vi "Cmd.Echo.vi"(6 "Timeout [ms] (1000)":i32=1000, 8 "error in":errorcluster, 10 "String":string="echoo", 11 "cID in":refnum<k5>) -> (0 "error out":errorcluster, 3 "cID out":refnum<k5>)   [LabVIEW 2016]
panel:
  out "debug":string
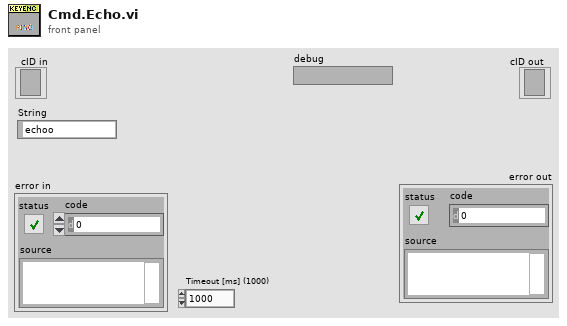
[diagram p1: front panel]
types:
  T1 = enum16{"Standard", "Buffered", "CRLF", "Immediate"}
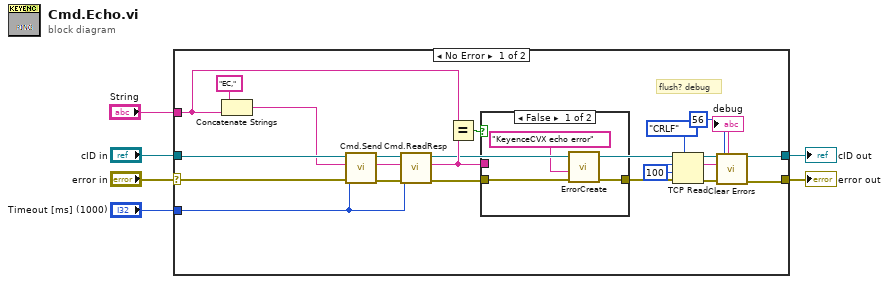
[diagram p0: block diagram]
diagram:
  n1 = case shown="No Error" "error in" {
    selector: "error in" -> [w25 w31]
    tunnel: "Timeout [ms] (1000)" -> [w22 _]
    tunnel: "cID in" -> [w26 w32]
    tunnel: [w14 w32] -> w3
    tunnel: [w11 w31] -> w2
    tunnel: "String" -> [w19 _]
    frame No Error {
      w7 = 100 ("timeout ms (25000)")
      # "flush? debug"
      n2 = Concatenate Strings("EC,", w19) -> (w20:string)
      n3 = call "Cmd.Send.vi"("error in (no error)"=w25, "Timeout [ms] (1000)"=w22, "Command"=w20, "connection ID"=w26) -> ("error out"=w23:errorcluster, "connection ID out"=w24:refnum<k5>)  [unwired: 6 in]
      n4 = call "Cmd.ReadResp.vi"("error in (no error)"=w23, "Timeout [ms] (1000)"=w22, "Request"=w20, "connection ID"=w24) -> ("error out"=w18:errorcluster, "ResponseParameters"=w16:string, "connection ID out"=w15:refnum<k5>)  [unwired: 5 in]
      n5 = Equal?(x=w19, y=w16) -> (x = y?=w17:bool)
      n6 = case shown="False" w17 {
        tunnel: w18 -> [w29 w30]
        tunnel: [w28 w30] -> w13
        tunnel: w16 -> [_ _]
        frame False {
          n7 = call "ErrorCreate.vi"("error in (no error)"=w29, "ErrorMessage"="KeyenceCVX echo error") -> ("error out"=w28:errorcluster)  [unwired: 9 in]
        }
        frame True {
        }
      }
      n8 = TCP Read(connection ID=w15, bytes to read=w7, error in (no error)=w13, 7:T1."CRLF" ("mode (standard)"), 9:w7) -> (connection ID out=w14:refnum<k5>, data out=→"debug":string, error out=w12:errorcluster)
      n9 = call <vilib>:"Clear Errors.vi"("error in (no error)"=w12, "specific error code to clear (0: all)"=56) -> ("error out"=w11:errorcluster)  [unwired: 4 in, 1 out]
    }
    frame Error {
    }
  }
  "cID out" <- w3
  "error out" <- w2
